vi "getGrating.vi"(8 "error in (no error)":errorcluster, 9 "Monochromator in":refnum<class "Monochromator.lvclass">, 11 "MonoState in":refnum<class "MonoState.lvclass">) -> (0 "error out":errorcluster, 1 "Monochromator out":refnum<class "Monochromator.lvclass">, 2 "GratingType":T1=enum."Red", 3 "MonoState out":refnum<class "MonoState.lvclass">)   [LabVIEW 2016, in "MonoState.lvclass"]
uses:
  MonoState.lvclass
  Typedefs/GratingType.ctl
  Monochromator/Monochromator.lvclass
  Monochromator/Monochromator.lvclass/Monochromator.ctl
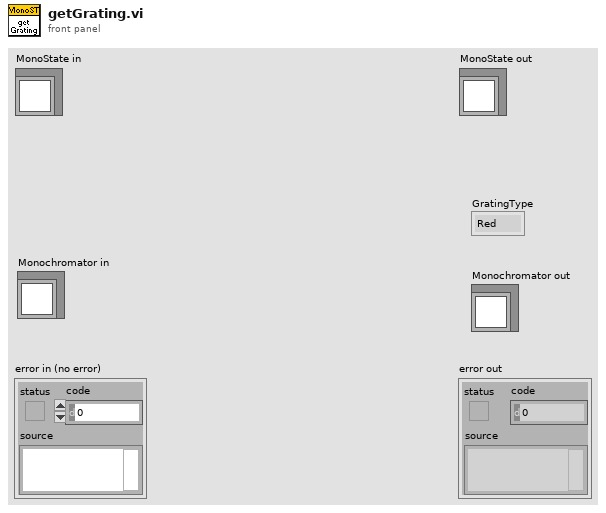
[diagram p1: front panel]
types:
  T1 = typedef "GratingType.ctl" = enum16{"Blue", "Red", "Mirror"}
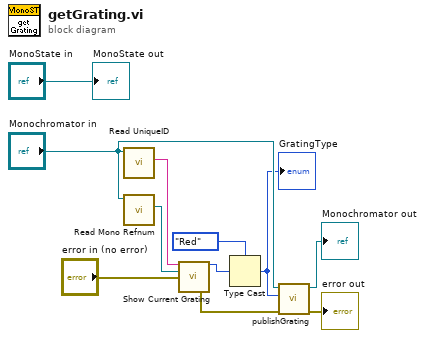
[diagram p0: block diagram]
diagram:
  n1 = call "Read UniqueID.vi"("Monochromator in"="Monochromator in") -> ("UniqueID"=w2:string)  [unwired: 8 in, 2 out]
  n2 = call "Read Mono Refnum.vi"("Monochromator in"="Monochromator in") -> ("Mono Refnum"=w3:refnum<k7>)  [unwired: 8 in, 2 out]
  n3 = call "Show Current Grating.vi"("UniqueID"=w2, "Refnum in"=w3, "error in (no error)"="error in (no error)") -> ("Grating Index"=w1:i32, "error out"=w5:errorcluster)  [unwired: 4 in, 7 out]
  n4 = Type Cast(type=GratingType."Red" ("GratingType 2"), x=w1) -> (*(type *) &x=w6:T1)
  "GratingType" <- w6
  n5 = call "publishGrating.vi"("error in (no error)"=w5, "GratingType"=w6, "Monochromator in"="Monochromator in") -> ("error out"=→"error out":errorcluster, "Monochromator out"=→"Monochromator out":refnum<class "Monochromator.lvclass">)  [unwired: 7 in]
  "MonoState out" <- "MonoState in"
